vi "2013_05_29 Pre-Clinical Main PWR Control.vi"() -> ()   [LabVIEW 2013]
uses:
  Pre-Clinical Type Def.ctl
  <vilib>/DAQmx/write.llb/DAQmx Write (Analog 1D DBL NChan 1Samp).vi
  <vilib>/DAQmx/write.llb/DAQmx Write (Counter Time 1Chan 1Samp).vi
  <vilib>/DAQmx/read.llb/DAQmx Read (Analog 1D Wfm NChan NSamp).vi
  <vilib>/DAQmx/miscellaneous.llb/DAQmx Fill In Error Info.vi
  <resource>/objmgr/daqmx.rc
panel:
  in  "PWM":dbl(slide)=100.0 min=0.0 max=100.0 step=1.0 scale=0.0..100.0 scale format="%#.2g"
  in  "error constant":dbl=4.5 step=0.0001
  out "Elapsed Time":dbl format="%<%H:%M:%S>t"
  in  "Reset RPM Max":bool
  out "RPM Max":u64
  in  "Manual/Voltage":bool
  in  "Step Mode":bool
  out "Target RPM":u64
  in  "Pwr Supply Port":refnum<visa-resource-name>="COM9"
  in  "Voltage":dbl(slide)=12.0 min=5.0 max=18.0 step=0.1 scale=5.0..18.0 scale format="%#.2g"
  in  "Off (s)":u32
  in  "On (s)":u32=120
  in  "On/Off":bool
  in  "Comments":string
  in  "Test ID and Serial #":string="default"
  in  "Motor":T1(ring)
  in  "Clear":bool
  in  "Record":bool=TRUE
  out "Error":bool
  out "XY Graph 3":cluster{"Array":dbl[], "Array":dbl[]}[](graph)
  in  "X axis":u16(ring)=5 items=["Elapsed Time (s)"=0, "Source Current (A)"=10, "Supply (V)"=4, "Supply Power (W)"=11, "RMS Current (A) 1"=1, "RMS Voltage (V) 1"=2, "Electrical Power (W)"=6, "ESC Efficiency (%)"=12, "Torque (mNm)"=5, "RPM"=3, "Mechanical Power(W)"=7, "Motor Efficiency (%)"=8]
  in  "Y axis":u16(ring)=3 items=["Elapsed Time (s)"=0, "Source Current (A)"=10, "Supply (V)"=4, "Supply Power (W)"=11, "RMS Current (A) 1"=1, "RMS Voltage (V) 1"=2, "Electrical Power (W)"=6, "ESC Efficiency (%)"=12, "Torque (mNm)"=5, "RPM"=3, "Mechanical Power(W)"=7, "Motor Efficiency (%)"=8]
  out "TotalSampPerChanAcquired":dbl
  out "AvailSampPerChan":u32
  out "XY Graph 2":cluster{"Array":dbl[], "Array":dbl[]}[](graph)
  out "Single Motor 2":waveform(dbl)[](graph)
  in  "Waveform":bool
  out "XY Graph":cluster{"Array":dbl[], "Array":dbl[]}(graph)
  out "error out":errorcluster
  in  "File Path":path=path "C:/Users/Will/Desktop/LabView/.lvm"
  in  "Motor 1":T2 {"ESC Eff" format="%#_3g%%"; "Supply (W)" format="%.3f"; "Mechanical (W)" format="%.3f"; "Motor Eff" format="%#_3g%%"; "Electrical (W)" format="%.3f"; "Torque (mNm)" format="%.3f"; "Time" format="%<%H:%M:%S>t"; "Supply (V)" format="%.2f"}
  out "loop time (ms)":u32
  in  "stop":bool
  # "Stopped"
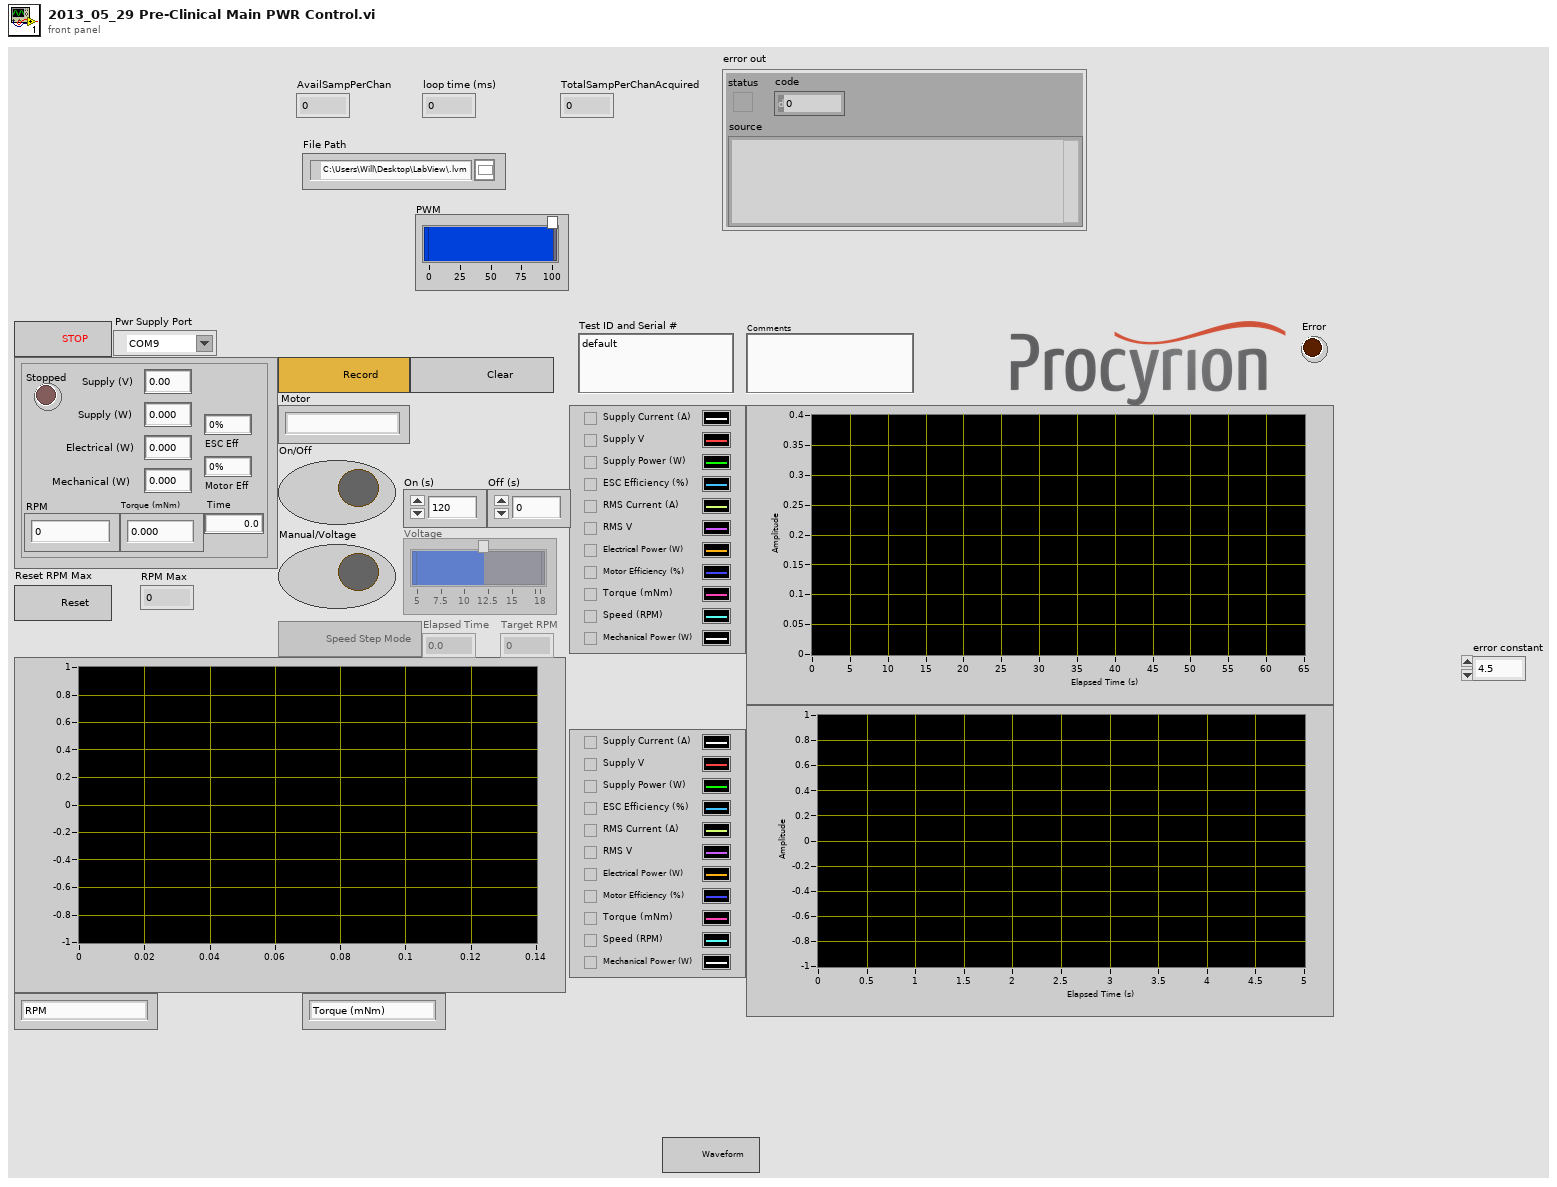
[diagram p1: front panel]
types:
  T1 = enum16{"", "Maxon EC6 6V", "Maxon EC4 6V", "FH 0620 6V", "FH 0620 12V", "FH 0427 6V K2540"}
  T2 = typedef "Pre-Clinical Type Def.ctl" = cluster{"Fail":bool, "RPM":u64, "Supply (V)":dbl, "Time":dbl, "Counter":dbl, "Torque (mNm)":dbl, "Electrical (W)":dbl, "Motor Eff":dbl, "Mechanical (W)":dbl, "Supply (W)":dbl, "ESC Eff":dbl}
  T3 = enum8{"Enabled", "Disabled", "Disabled and Grayed Out"}
  T4 = cluster{"Test ID and Serial #":string, "Comments":string, "Motor":enum16{"", "Maxon EC6 6V", "Maxon EC4 6V", "FH 0620 6V", "FH 0620 12V", "FH 0427 6V K2540"}, "Record":bool, "Clear":bool}
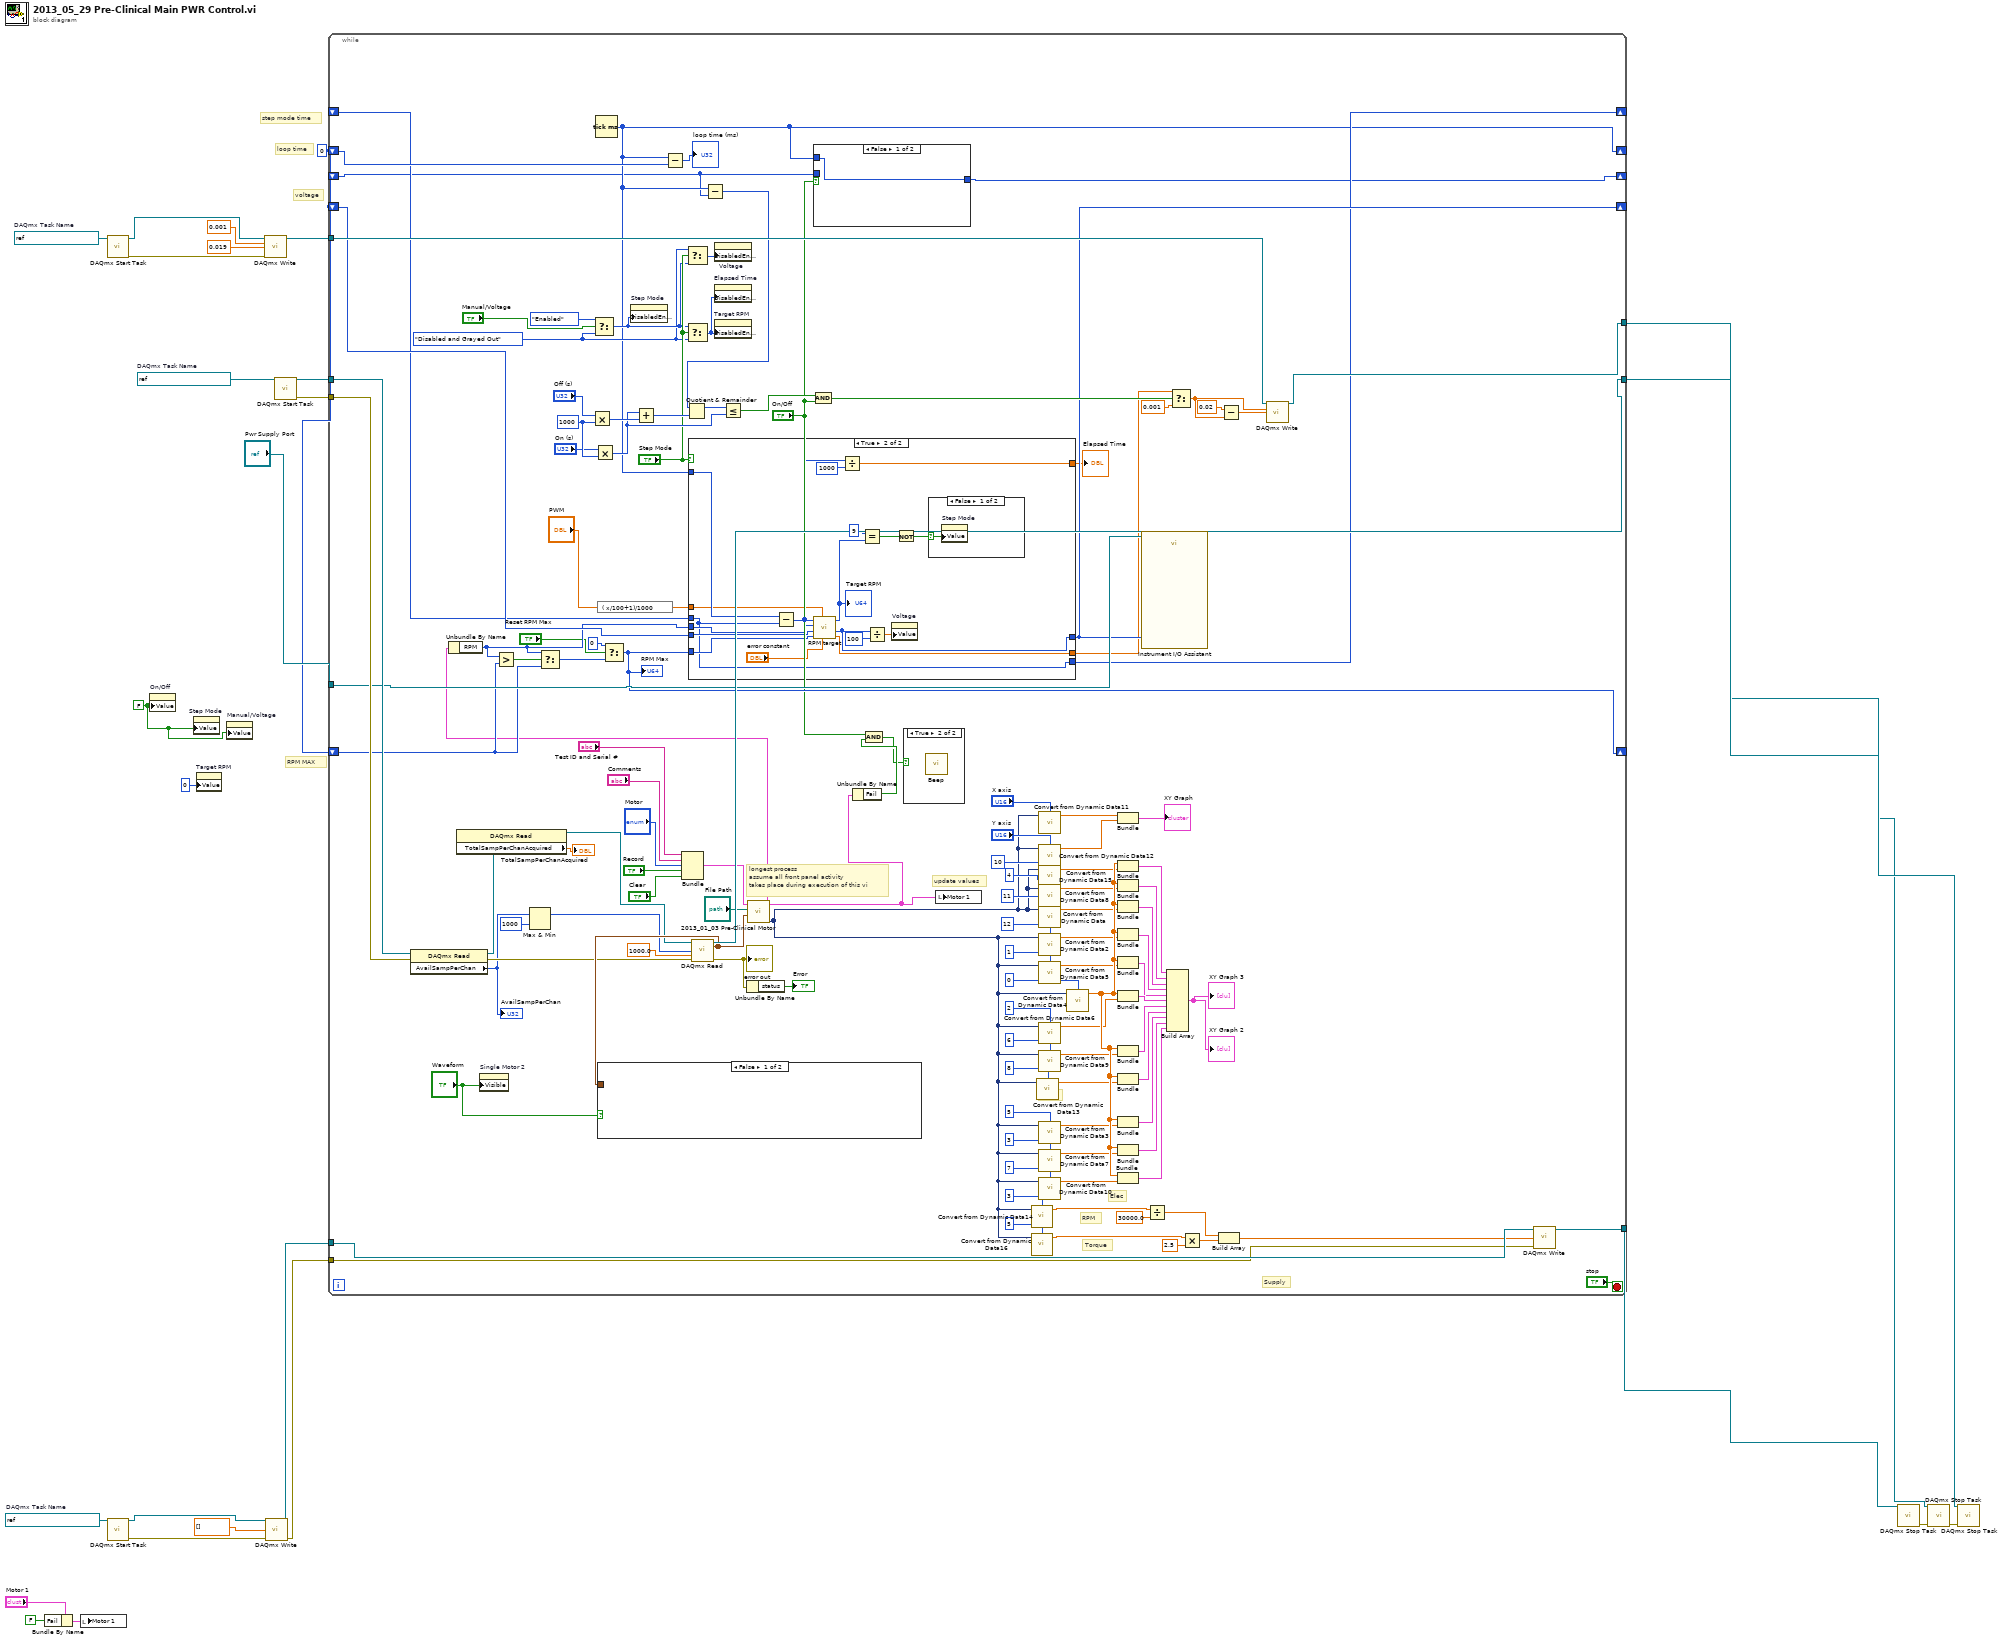
[diagram p0: block diagram]
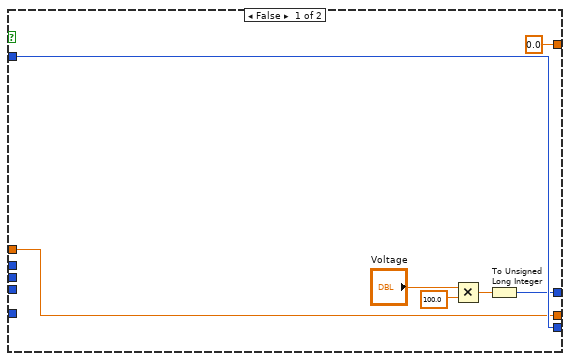
[diagram p4: hidden frame]
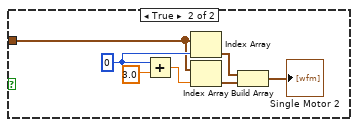
[diagram p6: hidden frame]
diagram:
  w2 = FALSE ("On/Off")
  w12 = refnum<k21> "Pre-Clinical ADI Out"  # DAQmx Task Name
  w3 = u32 0 ("millisecond timer value")
  w25 = refnum<k21> "Pre-Clinical PWM"  # DAQmx Task Name
  w13 = refnum<k21> "Pre-Clinical Acquire"  # DAQmx Task Name
  # "step mode time"
  # "RPM MAX"
  # "voltage"
  # "loop time"
  n1 = Bundle By Name(cluster="Motor 1", "Fail"=FALSE) -> (w14:T2)
  n2 = local write "Motor 1"(w14) -> ()
  n3 = call <vilib>:"DAQmx Start Task.vi"("task/channels in"=w25) -> ("task out"=w23:refnum<k21>, "error out"=w22:errorcluster)  [unwired: 13 in]
  n4 = call <vilib>:"DAQmx Start Task.vi"("task/channels in"=w12) -> ("task out"=w11:refnum<k21>, "error out"=w10:errorcluster)  [unwired: 13 in]
  n5 = property on="On/Off" class="Bool (strict)"("Value"=w2) -> ()  [unwired: 2 in, 2 out]
  n6 = property on="Step Mode" class="Bool (strict)"("Value"=w2) -> ()  [unwired: 2 in, 2 out]
  n7 = property on="Target RPM" class="DigNum (strict)"("Value"=u64 0 ("Target RPM")) -> ()  [unwired: 2 in, 2 out]
  n8 = property on="Manual/Voltage" class="Bool (strict)"("Value"=w2) -> ()  [unwired: 2 in, 2 out]
  n9 = call-poly <vilib>:"DAQmx Write.vi"("task/channels in"=w23, "high time"=0.001 ("data"), "low time"=0.019 ("data"), "error in"=w22) -> ("task out"=w24:refnum<k21>)  [unwired: 9 in, 2 out]
  n10 = call-poly <vilib>:"DAQmx Write.vi"("task/channels in"=w11, "data"=dbl[] [], "error in"=w10) -> ("task out"=w9:refnum<k21>, "error out"=w7:errorcluster)  [unwired: 10 in, 1 out]
  n11 = call <vilib>:"DAQmx Start Task.vi"("task/channels in"=w13) -> ("task out"=w27:refnum<k21>, "error out"=w17:errorcluster)  [unwired: 13 in]
  n12 = while {
    tunnel: w27 -> [w131]
    tunnel: [w147] -> w26
    tunnel: w17 -> [w129]
    shift-right: [w35] -> _
    shift-left: w3 -> [w151]
    tunnel: w24 -> [w149]
    tunnel: [w148] -> w21
    tunnel: w9 -> [w94]
    tunnel: w7 -> [w87]
    tunnel: [w86] -> w6
    tunnel: "Pwr Supply Port" -> [w58]
    shift-right: [w57] -> _
    shift-left: w3 -> [w56]
    shift-right: [w46] -> _
    shift-left: w3 -> [w53]
    shift-right: [w52] -> _
    shift-left: _ -> [w51]
    shift-right: [w36] -> _
    shift-left: _ -> [w34]
    stop <- "stop" stop-if-true
    w40 = T3."Disabled and Grayed Out" ("Disabled")
    w65 = u32 1000 ("y")
    # "Torque"
    # "RPM"
    # "Mech"
    # "Elec"
    # "Supply"
    # "update values"
    # "longest process\nassume all front panel activity\ntakes place during execution of this vi"
    n13 = property class="DAQmx Read"(reference=w131, error in=w129) -> (reference out=w127:refnum<k21>, error out=w128:errorcluster, "AvailSampPerChan"=w123:u32)
    "AvailSampPerChan" <- w123
    n14 = property class="DAQmx Read"(reference=w127) -> (reference out=w126:refnum<k21>, "TotalSampPerChanAcquired"=→"TotalSampPerChanAcquired":dbl)  [unwired: 1 in, 1 out]
    n15 = property on="Single Motor 2" class="WFGraph (strict)"("Visible"="Waveform") -> ()  [unwired: 2 in, 2 out]
    n16 = Max & Min(x=w123, y=1000 ("number of samples per channel")) -> (max(x,y)=w122:u32)  [unwired: 1 out]
    n17 = Multiply(x="Off (s)", y=w65) -> (x*y=w67:u32)
    n18 = Select(t=T3."Enabled" ("Disabled"), s="Manual/Voltage", f=w40) -> (s? t:f=w41:T3)
    n19 = Multiply(x="On (s)", y=w65) -> (x*y=w62:u32)
    n20 = Tick Count (ms)() -> (millisecond timer value=w35:u32)
    n21 = expression code="( x/100+1)/1000"("PWM") -> (w38:dbl)
    n22 = property on="Step Mode" class="Bool (strict)"("DisabledEnum"=w41) -> ()  [unwired: 2 in, 2 out]
    n23 = Add(x=w62, y=w67) -> (x+y=w66:u32)
    n24 = Subtract(x=w35, y=w151) -> (x-y=→"loop time (ms)":u32)
    n25 = Bundle("Test ID and Serial #"="Test ID and Serial #", "Comments"="Comments", "Motor"="Motor", "Record"="Record", "Clear"="Clear") -> (w59:T4)  [unwired: 1 in]
    n26 = Select(t=w40, s="Step Mode", f=w41) -> (s? t:f=w43:T3)
    n27 = Select(t=w41, s="Step Mode", f=w40) -> (s? t:f=w39:T3)
    n28 = call-poly <vilib>:"DAQmx Read.vi"("task/channels in"=w126, "number of samples per channel"=w122, "timeout"=1000.0, "error in"=w128) -> ("task out"=w147:refnum<k21>, "data"=w146:waveform(dbl)[], "error out"=w95:errorcluster)  [unwired: 9 in]
    "error out" <- w95
    n29 = case shown="False" "Waveform" {
      tunnel: w146 -> [_ w185]
      frame False {
      }
      frame True {
        w186 = 0 ("index")
        n30 = Add(x=w186, y=3.0) -> (x+y=w184:dbl)
        n31 = Index Array(array=w185, index=w186) -> (element=w183:waveform(dbl))
        n32 = Index Array(array=w185, index=w184) -> (element=w182:waveform(dbl))
        n33 = Build Array(w183, w182) -> (→"Single Motor 2":waveform(dbl)[])
      }
    }
    n34 = Subtract(x=w35, y=w34) -> (x-y=w33:u32)
    n35 = Quotient & Remainder(x=w33, y=w66) -> (x-y*floor(x/y)=w68:u32)  [unwired: 1 out]
    n36 = property on="Voltage" class="Slide (strict)"("DisabledEnum"=w43) -> ()  [unwired: 2 in, 2 out]
    n37 = property on="Elapsed Time" class="DigNum (strict)"("DisabledEnum"=w39) -> ()  [unwired: 2 in, 2 out]
    n38 = property on="Target RPM" class="DigNum (strict)"("DisabledEnum"=w39) -> ()  [unwired: 2 in, 2 out]
    n39 = Less Or Equal?(x=w68, y=w62) -> (x <= y?=w61:bool)
    n40 = Unbundle By Name(w95) -> ("status"=→"Error":bool)
    n41 = call "2013_01_03 Pre-Clinical Motor.vi"("data"=w146, "File Path"="File Path", "cluster"=w59) -> ("Final Out"=w90:dynamicdata, "Motor Typedef Out"=w31:T2)  [unwired: 7 in]
    n42 = Unbundle By Name(w31) -> ("RPM"=w54:u64)
    n43 = Greater?(x=w54, y=w53) -> (0:w55:bool)
    n44 = Select(t=w54, s=w55, f=w53) -> (s? t:f=w47:u64)
    n45 = Select(t=u64 0, s="Reset RPM Max", f=w47) -> (s? t:f=w46:u64)
    "RPM Max" <- w46
    n46 = case shown="True" "Step Mode" {
      tunnel: [w158 w165] -> w57
      tunnel: w56 -> [_ w179]
      tunnel: w54 -> [_ w178]
      tunnel: w46 -> [_ w177]
      tunnel: w35 -> [w161 w174]
      tunnel: [w161 w173] -> w52
      tunnel: w51 -> [_ w173]
      tunnel: [0.0 w169] -> w44
      tunnel: w38 -> [w155 w167]
      tunnel: [w155 w166] -> w37
      frame False {
        n47 = Multiply(x="Voltage", y=100.0) -> (x*y=w157:dbl)
        n48 = To Unsigned Long Integer(number=w157) -> (unsigned 32bit integer=w158:u32)
      }
      frame True {
        n49 = Subtract(x=w174, y=w173) -> (x-y=w171:u32)
        n50 = call "RPM target.vi"("error constant"="error constant", "PWM IN"=w167, "RPM MAX"=w177, "Voltage IN"=w179, "RPM IN"=w178, "elapsed ms"=w171) -> ("PWM"=w166:dbl, "Voltage OUT"=w165:u32, "New Target RPM"=w162:u64)  [unwired: 3 in]
        "Target RPM" <- w162
        n51 = Divide(x=w171, y=u32 1000) -> (x/y=w169:dbl)
        n52 = Equal?(x=u64 9, y=w162) -> (x = y?=w175:bool)
        n53 = Divide(x=w165, y=u32 100) -> (x/y=w163:dbl)
        n54 = property on="Voltage" class="Slide (strict)"("Value"=w163) -> ()  [unwired: 2 in, 2 out]
        n55 = Not(x=w175) -> (.not. x?=w172:bool)
        n56 = case shown="False" w172 {
          selector: w172 -> [w180 _]
          frame False {
            n57 = property on="Step Mode" class="Bool (strict)"("Value"=w180) -> ()  [unwired: 2 in, 2 out]
          }
          frame True {
          }
        }
      }
    }
    "Elapsed Time" <- w44
    n58 = And(x=w61, y="On/Off") -> (x .and. y?=w60:bool)
    n59 = case shown="False" "On/Off" {
      tunnel: [w153 w154] -> w36
      tunnel: w34 -> [_ w154]
      tunnel: w35 -> [w153 _]
      frame False {
      }
      frame True {
      }
    }
    n60 = Unbundle By Name(w31) -> ("Fail"=w30:bool)
    n61 = And(x="On/Off", y=w30) -> (x .and. y?=w28:bool)
    n62 = case shown="True" w28 {
      frame False {
      }
      frame True {
        n63 = call <vilib>:"Beep.vi"() -> ()  [unwired: 12 in]
      }
    }
    n64 = local write "Motor 1"(w31) -> ()
    n65 = call "Convert from Dynamic Data14"("Dynamic Data Type"=w90, "Channel"=3) -> ("Scalar"=w84:dbl)  [unwired: 2 in]
    n66 = call "Convert from Dynamic Data16"("Dynamic Data Type"=w90, "Channel"=5) -> ("Scalar"=w79:dbl)  [unwired: 2 in]
    n67 = call "Convert from Dynamic Data13"("Dynamic Data Type"=w90, "Channel"=8) -> ("Array"=w97:dbl[])  [unwired: 2 in]
    n68 = call "Convert from Dynamic Data11"("Dynamic Data Type"=w90, "Channel"="X axis") -> ("Array"=w119:dbl[])  [unwired: 2 in]
    n69 = call "Convert from Dynamic Data12"("Dynamic Data Type"=w90, "Channel"="Y axis") -> ("Array"=w120:dbl[])  [unwired: 2 in]
    n70 = call "Convert from Dynamic Data15"("Dynamic Data Type"=w90, "Channel"=10) -> ("Array"=w117:dbl[])  [unwired: 2 in]
    n71 = call "Convert from Dynamic Data8"("Dynamic Data Type"=w90, "Channel"=4) -> ("Array"=w103:dbl[])  [unwired: 2 in]
    n72 = call "Convert from Dynamic Data"("Dynamic Data Type"=w90, "Channel"=11) -> ("Array"=w102:dbl[])  [unwired: 2 in]
    n73 = call "Convert from Dynamic Data2"("Dynamic Data Type"=w90, "Channel"=12) -> ("Array"=w101:dbl[])  [unwired: 2 in]
    n74 = call "Convert from Dynamic Data5"("Dynamic Data Type"=w90, "Channel"=1) -> ("Array"=w100:dbl[])  [unwired: 2 in]
    n75 = call "Convert from Dynamic Data6"("Dynamic Data Type"=w90, "Channel"=2) -> ("Array"=w99:dbl[])  [unwired: 2 in]
    n76 = call "Convert from Dynamic Data9"("Dynamic Data Type"=w90, "Channel"=6) -> ("Array"=w116:dbl[])  [unwired: 2 in]
    n77 = call "Convert from Dynamic Data3"("Dynamic Data Type"=w90, "Channel"=5) -> ("Array"=w92:dbl[])  [unwired: 2 in]
    n78 = call "Convert from Dynamic Data7"("Dynamic Data Type"=w90, "Channel"=3) -> ("Array"=w91:dbl[])  [unwired: 2 in]
    n79 = call "Convert from Dynamic Data10"("Dynamic Data Type"=w90, "Channel"=7) -> ("Array"=w98:dbl[])  [unwired: 2 in]
    n80 = call "Convert from Dynamic Data4"("Dynamic Data Type"=w90, "Channel"=0) -> ("Array"=w118:dbl[])  [unwired: 2 in]
    n81 = Bundle("Array"=w119, "Array"=w120) -> (→"XY Graph":cluster{"Array":dbl[], "Array":dbl[]})  [unwired: 1 in]
    n82 = Bundle("Array"=w118, "Array"=w117) -> (w135:cluster{"Array":dbl[], "Array":dbl[]})  [unwired: 1 in]
    n83 = Bundle("Array"=w118, "Array"=w103) -> (w136:cluster{"Array":dbl[], "Array":dbl[]})  [unwired: 1 in]
    n84 = Bundle("Array"=w118, "Array"=w102) -> (w137:cluster{"Array":dbl[], "Array":dbl[]})  [unwired: 1 in]
    n85 = Bundle("Array"=w118, "Array"=w101) -> (w138:cluster{"Array":dbl[], "Array":dbl[]})  [unwired: 1 in]
    n86 = Bundle("Array"=w118, "Array"=w100) -> (w139:cluster{"Array":dbl[], "Array":dbl[]})  [unwired: 1 in]
    n87 = Bundle("Array"=w118, "Array"=w99) -> (w140:cluster{"Array":dbl[], "Array":dbl[]})  [unwired: 1 in]
    n88 = Bundle("Array"=w118, "Array"=w116) -> (w141:cluster{"Array":dbl[], "Array":dbl[]})  [unwired: 1 in]
    n89 = Bundle("Array"=w118, "Array"=w97) -> (w142:cluster{"Array":dbl[], "Array":dbl[]})  [unwired: 1 in]
    n90 = Bundle("Array"=w118, "Array"=w92) -> (w144:cluster{"Array":dbl[], "Array":dbl[]})  [unwired: 1 in]
    n91 = Bundle("Array"=w118, "Array"=w91) -> (w143:cluster{"Array":dbl[], "Array":dbl[]})  [unwired: 1 in]
    n92 = Bundle("Array"=w118, "Array"=w98) -> (w133:cluster{"Array":dbl[], "Array":dbl[]})  [unwired: 1 in]
    n93 = call "Instrument I/O Assistant"("Session In"=w58, "voltage"=w57) -> ()  [unwired: 24 in, 2 out]
    n94 = Divide(x=w84, y=30000.0) -> (x/y=w83:dbl)
    n95 = Build Array(w135, w136, w137, w138, w139, w140, w141, w142, w144, w143, w133) -> (→"XY Graph 2" →"XY Graph 3":cluster{"Array":dbl[], "Array":dbl[]}[])
    n96 = Select(t=w37, s=w60, f=0.001) -> (s? t:f=w70:dbl)
    n97 = Multiply(x=w79, y=2.5) -> (x*y=w80:dbl)
    n98 = Build Array(w83, w80) -> (w82:dbl[])
    n99 = Subtract(x=0.02 ("y"), y=w70) -> (x-y=w71:dbl)
    n100 = call-poly <vilib>:"DAQmx Write.vi"("task/channels in"=w149, "high time"=w70, "low time"=w71) -> ("task out"=w148:refnum<k21>)  [unwired: 10 in, 2 out]
    n101 = call-poly <vilib>:"DAQmx Write.vi"("task/channels in"=w94, "data"=w82, "error in"=w87) -> ("task out"=w86:refnum<k21>)  [unwired: 10 in, 2 out]
  }
  n102 = call <vilib>:"DAQmx Stop Task.vi"("task/channels in"=w6) -> ("error out"=w5:errorcluster)  [unwired: 13 in, 1 out]
  n103 = call <vilib>:"DAQmx Stop Task.vi"("task/channels in"=w21, "error in"=w5) -> ("error out"=w20:errorcluster)  [unwired: 12 in, 1 out]
  n104 = call <vilib>:"DAQmx Stop Task.vi"("task/channels in"=w26, "error in"=w20) -> ()  [unwired: 12 in, 2 out]
